vi "AutoVars.vi"() -> ()   [LabVIEW 2015]
panel:
  out "ArmInitDone":bool
  out "ReqDriveSpeed":dbl=-1.0
  out "ReqManipPosition":dbl
  out "FailInitDone":bool
  out "ReqArmPosition":dbl=297.0
  out "FarLeft":bool=TRUE
  out "RampartFactor":bool
  out "DriveInitDone":bool=TRUE
  in  "AutoStateMachine":T1(ring)
  out "VarsReceived":bool=TRUE
  out "EstDegToTurn":dbl=37.0
  out "DistanceToDrive":dbl=-68000.0
  out "DirectionToTurn":dbl=1.0
  in  "Defense":T2(ring)
  in  "RobotStartingPosition":T3(ring)
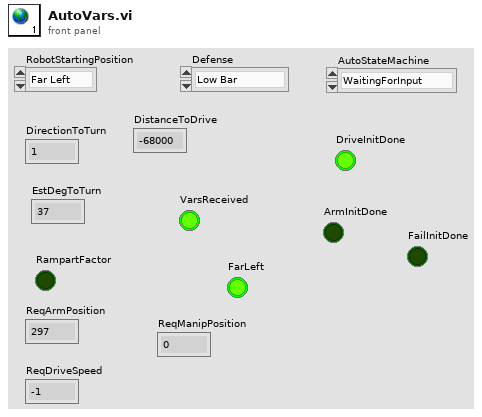
[diagram p1: front panel]
types:
  T1 = enum16{"WaitingForInput", "Driving", "TurnToTarget", "DriveMore", "Shoot", "End"}
  T2 = enum16{"Low Bar", "Ramparts", "Moat", "Rock Wall", "Rough Terrain", "Portcullis", "Cheval de Frise", "Drawbridge", "Sally Port"}
  T3 = enum16{"Far Left", "Pos 2", "Pos 3", "Pos 4", "Far Right"}
diagram:
